vi "read_commands.vi"(8 "error in (no error)":errorcluster, 11 "Path":path) -> (0 "error out":errorcluster, 3 "Command Array":string[](array[string]))   [LabVIEW 2015]
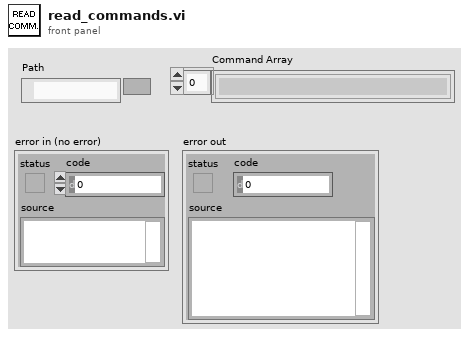
[diagram p1: front panel]
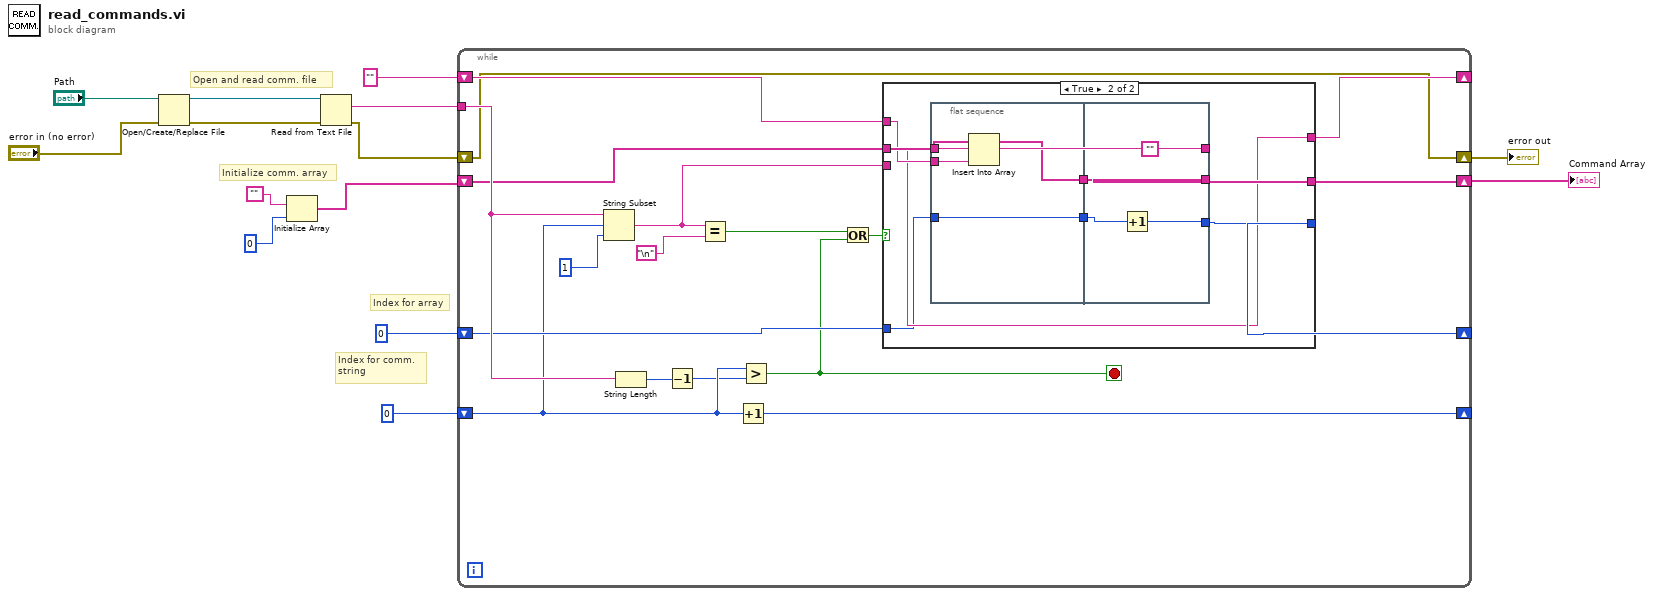
[diagram p0: block diagram]
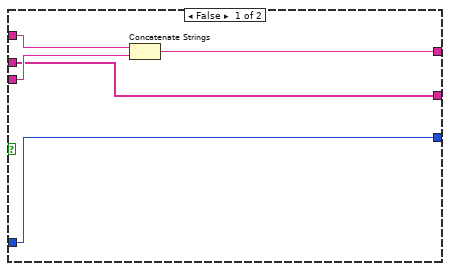
[diagram p2: hidden frame]
diagram:
  # "Open and read comm. file"
  # "Initialize comm. array"
  # "Index for comm.\nstring"
  # "Index for array"
  n1 = Open/Create/Replace File(file path (use dialog)="Path", error in="error in (no error)") -> (refnum out=w3:refnum<file>, error out=w4:errorcluster)  [unwired: 4 in, 1 out]
  n2 = Initialize Array("", 0) -> (w8:string[])
  n3 = Read from Text File(file (use dialog)=w3, error in=w4) -> (text=w13:string, error out=w12:errorcluster)  [unwired: 2 in, 2 out]
  n4 = while {
    tunnel: w13 -> [w31]
    shift-right: [w21] -> _
    shift-left: 0 -> [w20]
    shift-right: [w27] -> _
    shift-left: "" -> [w28]
    shift-right: [w25] -> w1
    shift-left: w8 -> [w26]
    shift-right: [w23] -> _
    shift-left: 0 -> [w24]
    shift-right: [w22] -> w2
    shift-left: w12 -> [w22]
    stop <- w15 stop-if-true
    n5 = String Subset(string=w31, offset (0)=w20, length (rest)=1) -> (substring=w29:string)
    n6 = String Length(string=w31) -> (length=w19:i32)
    n7 = Decrement(x=w19) -> (x-1=w18:i32)
    n8 = Equal?(x=w29, y="\n") -> (x = y?=w16:bool)
    n9 = Increment(x=w20) -> (x+1=w21:i32)
    n10 = Greater?(x=w20, y=w18) -> (0:w15:bool)
    n11 = Or(x=w16, y=w15) -> (x .or. y?=w17:bool)
    n12 = case shown="True" w17 {
      tunnel: w29 -> [w37 _]
      tunnel: [w36 w41] -> w27
      tunnel: w28 -> [w35 w44]
      tunnel: w26 -> [w34 w45]
      tunnel: [w34 w43] -> w25
      tunnel: w24 -> [w33 w40]
      tunnel: [w33 w38] -> w23
      frame False {
        n13 = Concatenate Strings(w35, w37) -> (w36:string)
      }
      frame True {
        n14 = flat-sequence {
          tunnel: w45 -> [w49]
          tunnel: w44 -> [w48]
          tunnel: [w47] -> w42
          tunnel: w40 -> [w46]
          tunnel: [w46] -> w39
          tunnel: [w53] -> w43
          tunnel: w42 -> [w53]
          tunnel: [""] -> w41
          tunnel: w39 -> [w51]
          tunnel: [w50] -> w38
          frame #0 {
            n15 = Insert Into Array(array=w49, new element=w48) -> (w47:string[])  [unwired: 1 in]
          }
          frame #1 {
            n16 = Increment(x=w51) -> (x+1=w50:i32)
          }
        }
      }
    }
  }
  "error out" <- w2
  "Command Array" <- w1
